vi "Read scrollbar.vi"(9 "Path in":refnum<class "Path.lvclass">) -> (3 "Path out":refnum<class "Path.lvclass">, 4 "scrollbar":bool)   [LabVIEW 2014, in "Path.lvclass"]
uses:
  Path.lvclass
  Path.lvclass/Path.ctl
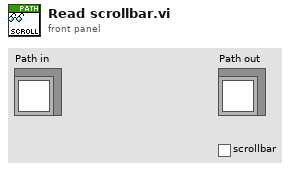
[diagram p1: front panel]
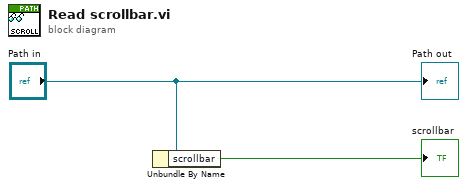
[diagram p0: block diagram]
diagram:
  n1 = Unbundle By Name("Path in") -> ("scrollbar"=→"scrollbar":bool)
  "Path out" <- "Path in"
